vi "Get Trigger ID.vi"(11 "STS Process in":refnum<class "STS Process.lvclass">) -> (2 "Trigger ID":u8, 3 "STS Process out":refnum<class "STS Process.lvclass">)   [LabVIEW 2019, in "TimingDRV Engine.lvlib" / "STS Process.lvclass"]
uses:
  STS Process.lvclass
  STS Process.lvclass/STS Process.ctl
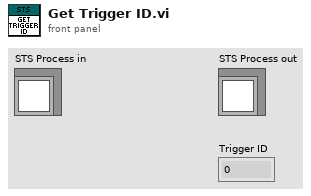
[diagram p1: front panel]
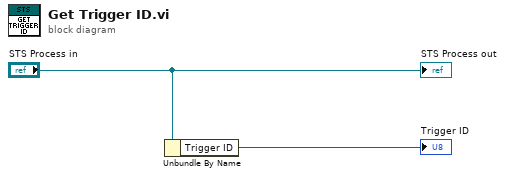
[diagram p0: block diagram]
diagram:
  n1 = Unbundle By Name("STS Process in") -> ("Trigger ID"=→"Trigger ID":u8)
  "STS Process out" <- "STS Process in"
